vi "Show-Hide Cursors.vi"(2 "Cursors On?(F)":bool, 3 "WFGraph Refnum":refnum<vi>) -> ()   [LabVIEW 2010]
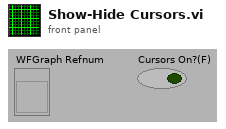
[diagram p1: front panel]
types:
  T1 = cluster{"Plot Area:Colors:FG Color":u32, "Plot Area:Colors:FG Color 2":u32}
  T2 = cluster{"Major Color":u32, "Plot Area:Colors:FG Color 2":u32}
  T3 = typedef "LVCursorListTypeDef.ctl" = cluster{"Name":string, "Color":u32, "Style":u8, "Point Style":u8, "Name Visible":bool, "Allow Drag":bool, "Cursor Mode":u32, "Plot":i32, "Index":i32, "Position":cluster{"X":dbl, "Y":dbl}, "X Scale":u32, "Y Scale":u32, "Watch Plots":i32[], "Watch All Plots":bool, "Plot Area":i32, "Label Offset":cluster{"X":dbl, "Y":dbl}}[]
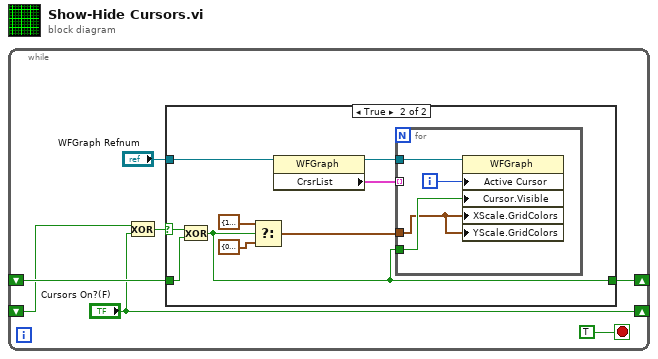
[diagram p0: block diagram]
diagram:
  n1 = while {
    shift-right: [w5] -> _
    shift-left: _ -> [w4]
    shift-right: ["Cursors On?(F)"] -> _
    shift-left: _ -> [w2]
    stop <- TRUE stop-if-true
    n2 = Exclusive Or(1:"Cursors On?(F)", 2:w2) -> (0:w1:bool)
    n3 = case shown="True" w1 {
      selector: w1 -> [_ w14]
      tunnel: "WFGraph Refnum" -> [_ w16]
      tunnel: [w8 w10] -> w5
      tunnel: w4 -> [w8 w13]
      frame False {
      }
      frame True {
        n4 = Exclusive Or(1:w13, 2:w14) -> (0:w10:bool)
        n5 = Select(t=T1 {"Plot Area:Colors:FG Color"=16777216, "Plot Area:Colors:FG Color 2"=16777216}, s=w10, f=cluster{"Major Color":u32, u32} {"Major Color"=0, 15198183} ("X Scale.Grid Colors")) -> (s? t:f=w11:T2)
        n6 = property on="Property Node" class="WFGraph"(reference=w16) -> (reference out=w15:refnum<vi>, "CrsrList"=w17:T3)  [unwired: 1 in, 1 out]
        n7 = for {
          tunnel: w17 -> [_] mode=indexing
          tunnel: w15 -> [w20]
          tunnel: w11 -> [w18]
          tunnel: w10 -> [w19]
          i -> [w21]
          n8 = property on="Property Node" class="WFGraph"(reference=w20, "Active Cursor"=w21, "Cursor.Visible"=w19, "XScale.GridColors"=w18, "YScale.GridColors"=w18) -> ()  [unwired: 1 in, 2 out]
        }
      }
    }
  }
